vi "Load Commiunication Error.vi"(8 "error in (no error)":errorcluster, 11 "main ref":T1) -> (0 "error out":errorcluster)   [LabVIEW 2025]
uses:
  controls/LAB-IQ UI Data.ctl
  Traction Loop/Traction Receipe Enum.ctl
  <vilib>/Analysis/baseanly.llb/Mean (DBL).vi
  <vilib>/Analysis/NI_AALBase.lvlib
panel:
  out "Load Comflg":bool
  out "OLD VAL":dbl
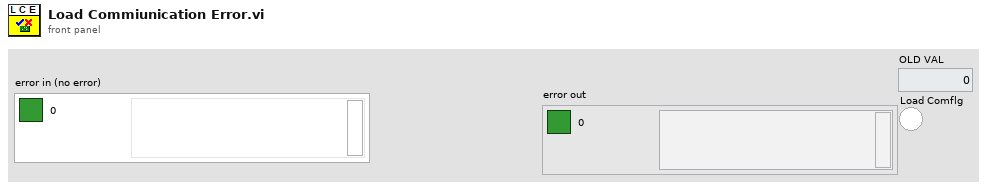
[diagram p1: front panel]
types:
  T1 = typedef "LAB-IQ UI Data.ctl" = cluster{"Main Home Screen":cluster{"GUI":refnum<vi>, "Platform Settings":refnum<vi>, "Configure":refnum<vi>, "Home":refnum<vi>, "EXIT":refnum<vi>, "service 2":refnum<vi>, "MainPage":refnum<vi>, "Analysis":refnum<vi>}, "Platform Settings":cluster{"mm/s  Surge":refnum<vi>, "Update Surge Speed":refnum<vi>, "Drive Error":refnum<vi>, "Disable Axis Jog Soft Limits":refnum<vi>, "mm/s  Sway":refnum<vi>, "Sway and Surge COM Status":refnum<vi>, "Heave COM Status":refnum<vi>, "Enable Platform":refnum<vi>, "Surge Forward Main":refnum<vi>, "Sway Right Main":refnum<vi>, "Sway Left Main":refnum<vi>, "Heave Down Main":refnum<vi>, "Heave Up main":refnum<vi>, "Update Sway Speed":refnum<vi>, "Update Heave Speed":refnum<vi>, "mm/s Heave":refnum<vi>, "mm/sec":refnum<vi>, "mm":refnum<vi>, "Surge Backward Main":refnum<vi>}, "Analysis Screen":cluster{"Analysis Home":refnum<vi>, "Surface Analysis":refnum<vi>, "Imaging":refnum<vi>, "Image Analysis":refnum<vi>, "Post Analysis":refnum<vi>}, "Config Screen":cluster{"Select Load Head":refnum<vi>, "Notes :":refnum<vi>, "FILE":refnum<vi>, "Sample ID :":refnum<vi>, "Operator ID :":refnum<vi>, "Operator Name :":refnum<vi>, "Auto":refnum<vi>}, "Motion Module":cluster{"zNL":refnum<vi>, "NL disp":refnum<vi>, "Rotary Tab":refnum<vi>, "Motion Direction:  3":refnum<vi>, "E.Velocity 2":refnum<vi>, "e.v/ssr 2":refnum<vi>, "Enter Fixed E.Velocity 2":refnum<vi>, "Enter Final SRR 2":refnum<vi>, "Enter initial SRR 2":refnum<vi>, "Enter Fixed SRR 2":refnum<vi>, "Enter the Final E.Velocity (m/s) 2":refnum<vi>, "Enter initial E.Velocity (m/s) 2":refnum<vi>, "Final Speed (RPM) 3":refnum<vi>, "Initial Speed (RPM) 2":refnum<vi>, "Enter the Final Velocity (m/s) 3":refnum<vi>, "Enter initial Velocity (m/s)  3":refnum<vi>, "Ramp Up 2":refnum<vi>, "TEST SELECTION":refnum<vi>, "SPEED SELECTION : ":refnum<vi>, "Angular Oscillation Set":refnum<vi>, "Traction":refnum<vi>, "Step Speed":refnum<vi>, "StepTable For Load-Speed":refnum<vi>, "StepTable For Speed":refnum<vi>, "Surge Forward MM":refnum<vi>, "Surge Backward MM":refnum<vi>, "M3 Image":refnum<vi>, "String 39":refnum<vi>, "Sway Left MM":refnum<vi>, "Sway Right MM":refnum<vi>, "Disable Axis Jog Soft Limits":refnum<vi>, "mm":refnum<vi>, "Heave Down MM":refnum<vi>, "Heave Up MM":refnum<vi>, "Wear Track Diameter (mm)":refnum<vi>, "Set WTD":refnum<vi>, "HomeScratch":refnum<vi>, "HomeRot":refnum<vi>, "PlaceModule":refnum<vi>, "Enter the Angle (Deg)":refnum<vi>, "Enter the Frequency (Hz)":refnum<vi>, "Motion Mode:":refnum<vi>, "LR Sway":refnum<vi>, "Rot Hor":refnum<vi>, "Scratch":refnum<vi>, "LR Cam":refnum<vi>, "MMBack":refnum<vi>, "MMNext":refnum<vi>, "Rot Ver":refnum<vi>, "Rotary Module Selection":refnum<vi>, "calculate rotary":refnum<vi>, "SPEED SELECTION : rotary":refnum<vi>, "Import 2":refnum<vi>, "Save 2":refnum<vi>, "File Path :  2":refnum<vi>, "String 45":refnum<vi>, "StepTable For Speed 3":refnum<vi>, "Enter the Speed(mm/sec)":refnum<vi>, "Enter the Speed(RPM)":refnum<vi>, "Enter Scratch Speed (mm/s):":refnum<vi>, "SwaySpeed Set":refnum<vi>, "Scartch Offset":refnum<vi>, "Motion type:":refnum<vi>, "HomeScratch 2":refnum<vi>, "Enter Scratch length (mm):":refnum<vi>, "Wear Track Diameter":refnum<vi>, "Rotary Speed Exced":refnum<vi>, "Scratch Mode":refnum<vi>, "No of Scratch":refnum<vi>}, "Environmental control":cluster{"Humidity  Status  3":refnum<vi>, "Low Temp  Status  2":refnum<vi>, "TK4 status 2":refnum<vi>, "Stage Temperature":refnum<vi>, "Sample Temperature":refnum<vi>, "Humidity (Amb)":refnum<vi>, "Clear List":refnum<vi>, "Add to list":refnum<vi>, "Wear":refnum<vi>, "Vibration":refnum<vi>, "Humidity (Chamber)":refnum<vi>, "Temperature (Chamber)":refnum<vi>, "ECR ":refnum<vi>, "Temperature (Amb)":refnum<vi>, "Microphone":refnum<vi>, "Acoustic Emission 3":refnum<vi>, "SNext":refnum<vi>, "APBack":refnum<vi>, "Enter the Temperature (°C):":refnum<vi>, "Enter the Stage \nTemperature (°C):":refnum<vi>, "Enter the Humidity (%Rh):":refnum<vi>, "Low Temp":refnum<vi>, "High Temp":refnum<vi>, "Humidity":refnum<vi>, "Sensors Picked":refnum<vi>}, "About Screen":cluster{"Password":refnum<vi>, "Home Service":refnum<vi>, "Advanced Setting":refnum<vi>, "About Tab":refnum<vi>, "ECR Port:":refnum<vi>, "Ramp Port:":refnum<vi>, "Installation/Replacement completed":refnum<vi>, "Loahead":refnum<vi>, "Heave and Surge COM Port:":refnum<vi>, "Sway COM Port:":refnum<vi>, "Temp Modbus:":refnum<vi>, "Humidity Port:":refnum<vi>, "Edit Gain Constants":refnum<vi>, "Save Gain Constants":refnum<vi>}, "Main Screen":cluster{"Main Screen Tab":refnum<vi>, "Angle and Frequency":refnum<vi>, "Stroke (mm)":refnum<vi>, "Angle (Deg)":refnum<vi>, "Main Speed Tab":refnum<vi>, "MTM MOTOR DISPLAY":refnum<vi>, "Disc Speed (m/sec)":refnum<vi>, "Ball Speed (m/sec)":refnum<vi>, "Disc Speed (RPM)":refnum<vi>, "Ball Speed (RPM)":refnum<vi>, "SPEED TAB":refnum<vi>, "Speed (m/sec)":refnum<vi>, "Set Speed (m/sec)":refnum<vi>, "Speed (RPM)":refnum<vi>, "Set Speed":refnum<vi>, "Time Tab":refnum<vi>, "Time ( HH:MM:SS ) 2":refnum<vi>, "Test Duration":refnum<vi>, "Test Duration 4":refnum<vi>, "TEST CYCLE":refnum<vi>, "TOTAL CYCLES":refnum<vi>, "Set Load (N)":refnum<vi>, "Temp Tabs":refnum<vi>, "Heater":refnum<vi>, "TK4 status":refnum<vi>, "ChamberTemp":refnum<vi>, "SetTmp":refnum<vi>, "Controller  Status":refnum<vi>, "ChamberTemp 2":refnum<vi>, "SetTmp 2":refnum<vi>, "Controller  Status 2":refnum<vi>, "ChamberTemp 3":refnum<vi>, "SetTmp 3":refnum<vi>, "Cooling":refnum<vi>, "Load Communication":refnum<vi>, "Ambient \nTemperature":refnum<vi>, "HumCOMStatus":refnum<vi>, "Ambient\n Humidity":refnum<vi>, "Freq (Hz)":refnum<vi>, "Load En":refnum<vi>, "NLt":refnum<vi>, "zNL 2":refnum<vi>, "Humidity On":refnum<vi>, "humidity disp":refnum<vi>, "Set Humidity":refnum<vi>, "NL disp 2":refnum<vi>, "Humidity On 2":refnum<vi>, "humidity disp 2":refnum<vi>, "Set Humidity 2":refnum<vi>, "NL disp 3":refnum<vi>, "AppLoadSeq scratch":refnum<vi>, "Stop Scratch":refnum<vi>, "ClrLog":refnum<vi>, "Trip Log":refnum<vi>, "STOP":refnum<vi>, "Start Test":refnum<vi>, "Test status":refnum<vi>, "AR Led":refnum<vi>, "Data":refnum<vi>, "Health":refnum<vi>, "Sway COM Status":refnum<vi>, "Heave COM Status":refnum<vi>, "Grp Tab":refnum<vi>, "Sub Graph":refnum<vi>, "SD (mm)":refnum<vi>, "Siliding distance Reset Graph":refnum<vi>, "SDGp":refnum<vi>, "Humidity Reset Graph":refnum<vi>, "HumrGp":refnum<vi>, "Acoustic Emission (mV)":refnum<vi>, "Aqucostic Reset Graph":refnum<vi>, "gACQUOS":refnum<vi>, "ECR RESET":refnum<vi>, "ECR":refnum<vi>, "Temperature Reset":refnum<vi>, "Acoustic Emission (mV) 2":refnum<vi>, "Aqucostic Reset Graph 2":refnum<vi>, "gACQUOS 2":refnum<vi>, "ECR RESET 2":refnum<vi>, "ECR 2":refnum<vi>, "Temperature Reset 2":refnum<vi>, "Temperature (deg c)":refnum<vi>, "Speed Reset Graph":refnum<vi>, "Speed Tab":refnum<vi>, "MTM DISC  SPEED":refnum<vi>, "MTM BALL SPEED":refnum<vi>, "speed mm/sec":refnum<vi>, "Hymidity":refnum<vi>, "Humidity Disable trip":refnum<vi>, "CoF Trip  2":refnum<vi>, "Depth Trip":refnum<vi>, "Weart Deapth":refnum<vi>, "Depth Reset Graph":refnum<vi>, "Weart":refnum<vi>, "Depthz":refnum<vi>, "Depth (µm)":refnum<vi>, "WearGp":refnum<vi>, "NL Trip 2":refnum<vi>, "Load pid":refnum<vi>, "Load Disable Trip":refnum<vi>, "Load Reset Graph":refnum<vi>, "NL Display 4":refnum<vi>, "Main Chart 3":refnum<vi>, "BACK":refnum<vi>, "Depth Trip 2":refnum<vi>, "COF TRIP ":refnum<vi>, "Friction Force (N)":refnum<vi>, "FF Reset Graph":refnum<vi>, "FF Disable Trip":refnum<vi>, "FF TRIP":refnum<vi>, "COF Disable Trip":refnum<vi>, "COF Reset Graph":refnum<vi>, "Start Test Temp":refnum<vi>, "zFF":refnum<vi>, "Friction Force (N) Graph":refnum<vi>, "Coefficient of Friction":refnum<vi>, "Scratch Start Test":refnum<vi>, "FF Tab":refnum<vi>, "Cyclic Friction Force (N)":refnum<vi>, "CZ FF":refnum<vi>, "Cyclic Friction Force (N) Graph":refnum<vi>, "Cyclic Coefficient of Friction":refnum<vi>, "Cyclic FF TRIP":refnum<vi>, "Cyclic FF Disable Trip":refnum<vi>, "cyclic COF Disable Trip":refnum<vi>, "cyclic COF TRIP":refnum<vi>, "cyclic COF Reset Graph":refnum<vi>, "Cyclic FF Reset Graph":refnum<vi>, "Test Trip":refnum<vi>, "Multi Scratch Pass":refnum<vi>, "Scratch Start Recording":refnum<vi>}, "Loading":cluster{"Indentation":refnum<vi>, "Reference Sample":refnum<vi>, "Load Cell Communication Slide":refnum<vi>, "com 3":refnum<vi>, "com":refnum<vi>, "DecaForce COM Status":refnum<vi>, "Update":refnum<vi>, "Clear 3":refnum<vi>, "seq":refnum<vi>, "Stribeck table":refnum<vi>, "Stribeck Table  For loading":refnum<vi>, "Loading Mode":refnum<vi>, "Enter the Final Load (N)":refnum<vi>, "Enter the CoF Trip":refnum<vi>, "Enter the Friction Force Trip":refnum<vi>, "Enter the Normal load Trip":refnum<vi>, "Enter the Load  (N)":refnum<vi>, "KiloForce":refnum<vi>, "DecaForce ":refnum<vi>, "MicroForce":refnum<vi>, "LHBack":refnum<vi>, "LHNext":refnum<vi>, "Enter the Loading Rate (N/min)":refnum<vi>, "Message":refnum<vi>, "Warning 2":refnum<vi>, "SSP 0.75":refnum<vi>, "SSP 0.5":refnum<vi>, "SSP 0.3":refnum<vi>, "Warning":refnum<vi>, "gui GIF":refnum<vi>, "Communication is established":refnum<vi>, "AppLoad 4":refnum<vi>, "Multipoint":refnum<vi>, "Load Selection":refnum<vi>}, "PID":cluster{"Ramp MulFac":refnum<vi>, "pulses LoadDiffRamp(2..10)":refnum<vi>, "PulseControlRamp(diff<=3N)":refnum<vi>, "SetLoadDeadband(%) Load(0-10N)":refnum<vi>, "PID gains out delay (microForce)":refnum<vi>, "Ramp":refnum<vi>, "Gain 2":refnum<vi>, "pulses LoadDiff(2..10)":refnum<vi>, "pulses LoadDiff(11..50)":refnum<vi>, "PulseControl(diff<=3N)":refnum<vi>, "SetLoadDeadband(%)  2":refnum<vi>, "Dummy Run":refnum<vi>, "Vertical load (N)":refnum<vi>, "AutoTune":refnum<vi>, "Offset 3 ":refnum<vi>, "apply load":refnum<vi>, "Offset  3":refnum<vi>, "apply load 2":refnum<vi>, "Enter ByPass Load":refnum<vi>, "reinit 3":refnum<vi>, "output range delay":refnum<vi>, "PID gains out delay":refnum<vi>, "Bypass Load":refnum<vi>, "pulsesSent":refnum<vi>, "pulses ":refnum<vi>, "actpid":refnum<vi>, "gFF Rot":refnum<vi>, "pulses LoadDiff(21..1000)":refnum<vi>, "Delay":refnum<vi>, "deadband":refnum<vi>}, "Config Parameters":cluster{"Tab Control 3":refnum<vi>, "Tab Control 19":refnum<vi>, "SAMPLES":refnum<vi>, "Re-initilaize":refnum<vi>, "Filter ON/OFF":refnum<vi>, "TracHomeSurgeOffsetCounts 10MM":refnum<vi>, "TracHomeSwayOffsetCounts 10MM":refnum<vi>, "Acoustic Emission:":refnum<vi>, "Apply Filter (FF)":refnum<vi>, "Filter% 2":refnum<vi>, "Apply Filter (Load)":refnum<vi>, "Filter% ":refnum<vi>, "Sway distance (mm)":refnum<vi>, "Surge distance (mm)":refnum<vi>, "DataSavingLoopDelay(ms)":refnum<vi>, "SAVE 2":refnum<vi>, "Enter Distance":refnum<vi>, "Sway Counts:":refnum<vi>, "Distance (mm): 3":refnum<vi>, "Surge Counts:":refnum<vi>, "Distance (mm): 2":refnum<vi>, "Distance (mm):":refnum<vi>, "Heave Counts:":refnum<vi>, "LRMHomeSurgeOffsetCounts":refnum<vi>, "LRMHomeSwayOffsetCounts":refnum<vi>, "TracHomeSurgeOffsetCounts 20MM":refnum<vi>, "TracHomeSwayOffsetCounts 20MM":refnum<vi>, "RotHomeSwayOffsetCounts":refnum<vi>, "RotHomeSurgeOffsetCounts":refnum<vi>, "Heave distance":refnum<vi>, "Zmm":refnum<vi>, "Heave Pulses/mm":refnum<vi>, "Surge Pulses/mm":refnum<vi>, "Sway Pulses/mm":refnum<vi>, "Heave Pitch":refnum<vi>, "Surge Pitch":refnum<vi>, "Sway Pitch":refnum<vi>, "Heave PPR":refnum<vi>, "Surge PPR":refnum<vi>, "Sway PPR":refnum<vi>, "Tab Control 5":refnum<vi>, "Tab Control 14":refnum<vi>, "Tab Control 26":refnum<vi>, "AE":refnum<vi>, "Heave Loop Delay":refnum<vi>, "Heave PID Speed":refnum<vi>, "Surge Jog Speed":refnum<vi>, "Heave Jog Speed":refnum<vi>, "Sway Loop Delay":refnum<vi>, "Sway PID Speed":refnum<vi>, "Sway Jog Speed":refnum<vi>, "DEPTH TRIP VALUE":refnum<vi>, "LOAD TRIP VALUE":refnum<vi>, "DEPTH TRIP   ENABLE":refnum<vi>, "LOAD TRIP  ENABLE":refnum<vi>, "CYCLIC FF TRIP VALUE":refnum<vi>, "FF TRIP VALUE":refnum<vi>, "CYCLIC CoF TRIP VALUE":refnum<vi>, "COF TRIP VALUE":refnum<vi>, "CYCLIC COF TRIP  ENABLE":refnum<vi>, "CYCLIC FF TRIP  ENABLE":refnum<vi>, "FF TRIP  ENABLE":refnum<vi>, "COF TRIP  ENABLE":refnum<vi>, "JOG TRIP LOAD VALUE (N)":refnum<vi>}, "Loading Com Port":cluster{"ClearAll":refnum<vi>, "Mz(Nm)":refnum<vi>, "My(Nm)":refnum<vi>, "Mx(Nm)":refnum<vi>, "Save Dwell":refnum<vi>, "Mx ":refnum<vi>, "My ":refnum<vi>, "Mz":refnum<vi>, "Fx(N)":refnum<vi>, "Fy(N)":refnum<vi>, "Fz(N)":refnum<vi>, "ZeroAll":refnum<vi>, "Acq Delay (ms)":refnum<vi>, "Burst Delay (ms)":refnum<vi>, "model":refnum<vi>, "SN":refnum<vi>, "FFx(N)":refnum<vi>, "Sensor IP":refnum<vi>, "Port":refnum<vi>, "FFy(N)":refnum<vi>, "Load(N)":refnum<vi>, "delete Handle":refnum<vi>, "Create Handle":refnum<vi>, "ft_data":refnum<vi>, "ft_range":refnum<vi>, "ft_data 2":refnum<vi>, "stop 6":refnum<vi>, "running_flag":refnum<vi>, "ft_udp_handle":refnum<vi>, "get-data-return":refnum<vi>, "get-range-return":refnum<vi>, "zero-return":refnum<vi>, "filter-return":refnum<vi>, "initial-return":refnum<vi>, "deleteHandle-result":refnum<vi>, "Load Cell Temp":refnum<vi>, "Load Cell":refnum<vi>}, "Heave AND Surge":cluster{"SURGE POSE":refnum<vi>, "error out Read":refnum<vi>, "HEAVE POSE":refnum<vi>, "State":refnum<vi>, "Homed":refnum<vi>, "Sequence ID":refnum<vi>, "error out Write":refnum<vi>, "faultCode":refnum<vi>, "Ack ID":refnum<vi>, "SPEED":refnum<vi>, "Distance":refnum<vi>, "Mode Command":refnum<vi>, "Heave and Surge Read":refnum<vi>, "Read Heave Temp":refnum<vi>, "Spare 15":refnum<vi>, "Spare 14":refnum<vi>, "Spare 13":refnum<vi>, "Spare 12":refnum<vi>, "Spare 11":refnum<vi>, "Spare 10":refnum<vi>, "Spare 9":refnum<vi>, "Spare 8":refnum<vi>, "Spare 7":refnum<vi>, "Spare 6":refnum<vi>, "Spare 5":refnum<vi>, "Spare 4":refnum<vi>, "Spare 2":refnum<vi>, "Spare 1":refnum<vi>, "Node Id":refnum<vi>, "Spare 3":refnum<vi>, "SPARE 4":refnum<vi>, "SPARE 3":refnum<vi>, "SPARE 2":refnum<vi>, "SPARE 1":refnum<vi>, "fwMajor":refnum<vi>, "fwMinor":refnum<vi>, "Manual Write":refnum<vi>, "Heave and Surge Write":refnum<vi>, "SPARE 5":refnum<vi>, "Reserved ":refnum<vi>, "SPARE 8":refnum<vi>, "SPARE 6":refnum<vi>, "SPARE 7":refnum<vi>, "SPARE 17":refnum<vi>, "SPARE 16":refnum<vi>, "SPARE 15":refnum<vi>, "SPARE 14":refnum<vi>, "SPARE 13":refnum<vi>, "SPARE 12":refnum<vi>, "SPARE 11":refnum<vi>, "SPARE 10":refnum<vi>, "SPARE 9":refnum<vi>, "System UPTIME":refnum<vi>, "Missed Packets":refnum<vi>, "faultCode Surge Right":refnum<vi>, "faultCode Surge Left":refnum<vi>, "faultCode Heave":refnum<vi>, "UPLINK HEAVE":refnum<vi>, "DOWNLINK HEAVE":refnum<vi>}, "New PID LOGIC":cluster{"Fine Tune Zone":refnum<vi>, "PID SDelay":refnum<vi>, "Max_pos_limit":refnum<vi>, "Min_pos_limit":refnum<vi>, "i_limit":refnum<vi>, "pct_scale":refnum<vi>, "Deadband":refnum<vi>, "Kd":refnum<vi>, "Ki":refnum<vi>, "Kp":refnum<vi>, "Current Position":refnum<vi>, "Set Load":refnum<vi>, "Current Load":refnum<vi>, "Pulse delta":refnum<vi>, "Init Step":refnum<vi>, "Max Step Linit":refnum<vi>, "min_deadband_floor":refnum<vi>, "dynamic_spindle_noise_scalar":refnum<vi>, "min_finetune_floor":refnum<vi>, "filter_alpha":refnum<vi>, "PID":refnum<vi>}, "SWAY ":cluster{"fwMajor":refnum<vi>, "Homed":refnum<vi>, "Rotary POSE":refnum<vi>, "State":refnum<vi>, "SWAY POSE":refnum<vi>, "Ack ID":refnum<vi>, "faultCode":refnum<vi>, "Node Id":refnum<vi>, "fwMinor":refnum<vi>, "Spare 6":refnum<vi>, "Spare 5":refnum<vi>, "Spare 4":refnum<vi>, "Spare 3":refnum<vi>, "Spare 2":refnum<vi>, "Spare 1":refnum<vi>, "Spare 7":refnum<vi>, "SPARE  5":refnum<vi>, "error out Write  SWAY ":refnum<vi>, "error out Read SWAY ":refnum<vi>, "Manual Write SWAY ":refnum<vi>, "SWAY WRITE":refnum<vi>, "SPARE  4":refnum<vi>, "SPARE  3":refnum<vi>, "SPARE 2":refnum<vi>, "SPARE 1":refnum<vi>, "Spare 15":refnum<vi>, "Spare 14":refnum<vi>, "Spare 13":refnum<vi>, "Spare 12":refnum<vi>, "Spare 11":refnum<vi>, "Spare 9":refnum<vi>, "Spare 8":refnum<vi>, "SPEED":refnum<vi>, "Distance":refnum<vi>, "Mode Command":refnum<vi>, "Sequence ID":refnum<vi>, "SWAY READ":refnum<vi>, "Spare 10":refnum<vi>, "Read SWAY Temp":refnum<vi>, "faultCode Sway ":refnum<vi>, "Missed Packets":refnum<vi>, "System UPTIME sway":refnum<vi>, "SPARE 6":refnum<vi>, "SPARE 7":refnum<vi>, "SPARE 9":refnum<vi>, "SPARE 11":refnum<vi>, "SPARE 10":refnum<vi>, "SPARE 8":refnum<vi>, "SPARE 13":refnum<vi>, "SPARE 12":refnum<vi>, "SPARE 17":refnum<vi>, "SPARE 16":refnum<vi>, "SPARE 15":refnum<vi>, "SPARE 14":refnum<vi>, "Reserved":refnum<vi>, "faultCode Rotary":refnum<vi>, "UPLINK SWAY":refnum<vi>, "DOWNLINK SWAY":refnum<vi>}, "Analysis Screen":cluster{"Analysis Home":refnum<vi>, "Refresh 2":refnum<vi>, "MEAN 4":refnum<vi>, "SD 4":refnum<vi>, "VARIANCE 4":refnum<vi>, "MEAN  3":refnum<vi>, "SD  3":refnum<vi>, "VARIANCE  3":refnum<vi>, "MEAN 2":refnum<vi>, "SD  2":refnum<vi>, "VARIANCE 2":refnum<vi>, "MEAN":refnum<vi>, "SD":refnum<vi>, "VARIANCE":refnum<vi>, "File 4 Discription":refnum<vi>, "OPEN 4":refnum<vi>, "File Name 4":refnum<vi>, "OPEN 3":refnum<vi>, "File 3 Discription":refnum<vi>, "File Name 3":refnum<vi>, "Y-AXIS":refnum<vi>, "X-AXIS":refnum<vi>, "XY Graph":refnum<vi>, "File Name 2":refnum<vi>, "File Name 1":refnum<vi>, "OPEN 2":refnum<vi>, "OPEN 1":refnum<vi>, "File 1 Discription ":refnum<vi>, "File 2 Discription":refnum<vi>, "Export":refnum<vi>, "File Format":refnum<vi>}, "Traction":cluster{"faultCode Traction 2":refnum<vi>, "faultCode Traction 1":refnum<vi>, "Missed Packets":refnum<vi>, "System UPTIME Traction":refnum<vi>, "SPARE 17":refnum<vi>, "SPARE 16":refnum<vi>, "SPARE 15":refnum<vi>, "SPARE 14":refnum<vi>, "SPARE 13":refnum<vi>, "SPARE 12":refnum<vi>, "SPARE 11":refnum<vi>, "SPARE 10":refnum<vi>, "SPARE 9":refnum<vi>, "SPARE 8":refnum<vi>, "SPARE 7":refnum<vi>, "SPARE 6":refnum<vi>, "Reserved":refnum<vi>, "SPARE  5":refnum<vi>, "Manual Write TRACTION":refnum<vi>, "TRACTION WRITE":refnum<vi>, "SPARE  4":refnum<vi>, "SPARE  3":refnum<vi>, "SPARE 2":refnum<vi>, "SPARE 1":refnum<vi>, "Spare 7":refnum<vi>, "Spare 6":refnum<vi>, "Spare 5":refnum<vi>, "Spare 4":refnum<vi>, "Spare 2":refnum<vi>, "Spare 1":refnum<vi>, "Node Id":refnum<vi>, "Read TRACTION Temp":refnum<vi>, "fwMinor":refnum<vi>, "fwMajor":refnum<vi>, "faultCode":refnum<vi>, "TRACTION POSE":refnum<vi>, "TRACTION POSE 2":refnum<vi>, "Homed":refnum<vi>, "State":refnum<vi>, "Ack ID":refnum<vi>, "SPEED":refnum<vi>, "Distance":refnum<vi>, "Mode Command":refnum<vi>, "Sequence ID":refnum<vi>, "error out Read TRACTION":refnum<vi>, "error out Write  TRACTION":refnum<vi>, "TRACTION READ":refnum<vi>, "Spare 3":refnum<vi>, "Downlink traction":refnum<vi>, "Uplink Traction":refnum<vi>}, "Traction reciepe":cluster{"SRR Sweep Range (%) Stribeck":refnum<vi>, "Traction Receipe":refnum<vi>, "Total Execution Time":refnum<vi>, "Total Steps":refnum<vi>, "Duration / Step (s)  Stribeck":refnum<vi>, "STRIBECK Fixed SRR List (%)":refnum<vi>, "Duration / Step (s) Traction":refnum<vi>, "SRR Sweep Range (%) traction":refnum<vi>, "Rolling Speed (mm/s)":refnum<vi>, "Temperature Stages (°C)":refnum<vi>, "Ball Load (N)":refnum<vi>, "Lubricant Name":refnum<vi>, "Profile File Name":refnum<vi>, "SET entrainment Velocity":refnum<vi>, "Test Array Size":refnum<vi>, "SRR INDEX [ STRIBECK]":refnum<vi>, "Stribeck Size":refnum<vi>, "SET SRR":refnum<vi>, "ELAPSED TIMER ":refnum<vi>, "BALL SET RPM":refnum<vi>, "DISC SET RPM":refnum<vi>, "SET LOAD":refnum<vi>, "TEMPERATURE READ":refnum<vi>, "SET TEMPERATURE":refnum<vi>, "Traction Size":refnum<vi>, "DISC SPEED (rpm)":refnum<vi>, "BALL SPEED (rpm)":refnum<vi>, "BALL WEAR TRACK":refnum<vi>, "DISC WEARTRACK":refnum<vi>, "SRR INDEX [ TRACTION]":refnum<vi>, "Start Index Type":refnum<vi>, "Enum - Menu":refnum<vi>, "Ball (mm/sec)":refnum<vi>, "Disc (mm/sec)":refnum<vi>}, "Traction Control":cluster{"HomeTraction":refnum<vi>, "Demo Mode Display":refnum<vi>, "Traction Message":refnum<vi>, "Traction Step Update Details":refnum<vi>, "Main Tab sequence for selection":refnum<vi>, "Ramp Tab":refnum<vi>, "e.v/ssr":refnum<vi>, "Enter Fixed E.Velocity":refnum<vi>, "Enter Final SRR":refnum<vi>, "Enter initial SRR":refnum<vi>, "Enter Fixed SRR":refnum<vi>, "Enter the Final E.Velocity (m/s)":refnum<vi>, "Enter initial E.Velocity (m/s)":refnum<vi>, "Ball WTD":refnum<vi>, "E.Velocity":refnum<vi>, "Enter the Final Velocity (m/s)":refnum<vi>, "Enter initial Velocity (m/s)":refnum<vi>, "Ramp Up   Disc":refnum<vi>, "Initial DiscSpeed (RPM)":refnum<vi>, "Final Speed (RPM) Ball":refnum<vi>, "Final Speed (RPM)":refnum<vi>, "Initial Speed (RPM) Ball":refnum<vi>, "Enter the Final Velocity (m/s) Ball":refnum<vi>, "Enter initial Velocity (m/s) Ball":refnum<vi>, "Ramp Up":refnum<vi>, "ExceedBallSpeed step":refnum<vi>, "ExceedDiscSpeed":refnum<vi>, "BallSpeed Exceed Indication":refnum<vi>, "Apply":refnum<vi>, "SPEED SELECTION : MTM":refnum<vi>, "SPEED SELECTION : MTM 2":refnum<vi>, "TEST SELECTION (MTM)":refnum<vi>, "MTM Test Selection":refnum<vi>, "File Path Tab":refnum<vi>, "File Path String":refnum<vi>, "Save":refnum<vi>, "Save  2":refnum<vi>, "Import ":refnum<vi>, "File Path :":refnum<vi>, "Step Sequence Indication Tab":refnum<vi>, "Step Sequence Indication":refnum<vi>, "Calculate Step":refnum<vi>, "StepTable":refnum<vi>, "ExceedDiscSpeed  Cinstant Speed":refnum<vi>, "ExceedBallSpeed Constant":refnum<vi>, "TEST SELECTION (MTM) 2":refnum<vi>, "SPEED SELECTION : MTM 3":refnum<vi>, "MTM Test Selection 2":refnum<vi>, "Enter the Speed (m/sec): ":refnum<vi>, "Enter the Speed (m/sec):  2":refnum<vi>, "Enter the Speed (RPM):":refnum<vi>, "Lower Spped ":refnum<vi>, "Upper":refnum<vi>, "Enter the Speed (RPM):Ball":refnum<vi>, "Disc Motion Direction: ":refnum<vi>, "Ball Motion Direction :":refnum<vi>, "Motion Mode: ":refnum<vi>, "Wear Track Diameter (mm) ":refnum<vi>, "Disc Speed Indicator":refnum<vi>, "ExceedBallSpeed":refnum<vi>}, "Acquostic":cluster{"Last Config Rejected ":refnum<vi>, "rx command count":refnum<vi>, "Current Filter Id":refnum<vi>, "Isolated Gain":refnum<vi>, "DAQ Status":refnum<vi>, "error out":refnum<vi>, "error in (no error)":refnum<vi>, "Uplink Packet":refnum<vi>, "data out":refnum<vi>, "Downlink Packet":refnum<vi>, "Signal Energy":refnum<vi>, "Amplitude db_AE":refnum<vi>, "Peak Amplitude":refnum<vi>, "AE Ring-Down Counts":refnum<vi>, "Gains":refnum<vi>, "Manual Write Acquostic":refnum<vi>}}
  T2 = enum8{"Enabled", "Disabled", "Disabled and Grayed Out"}
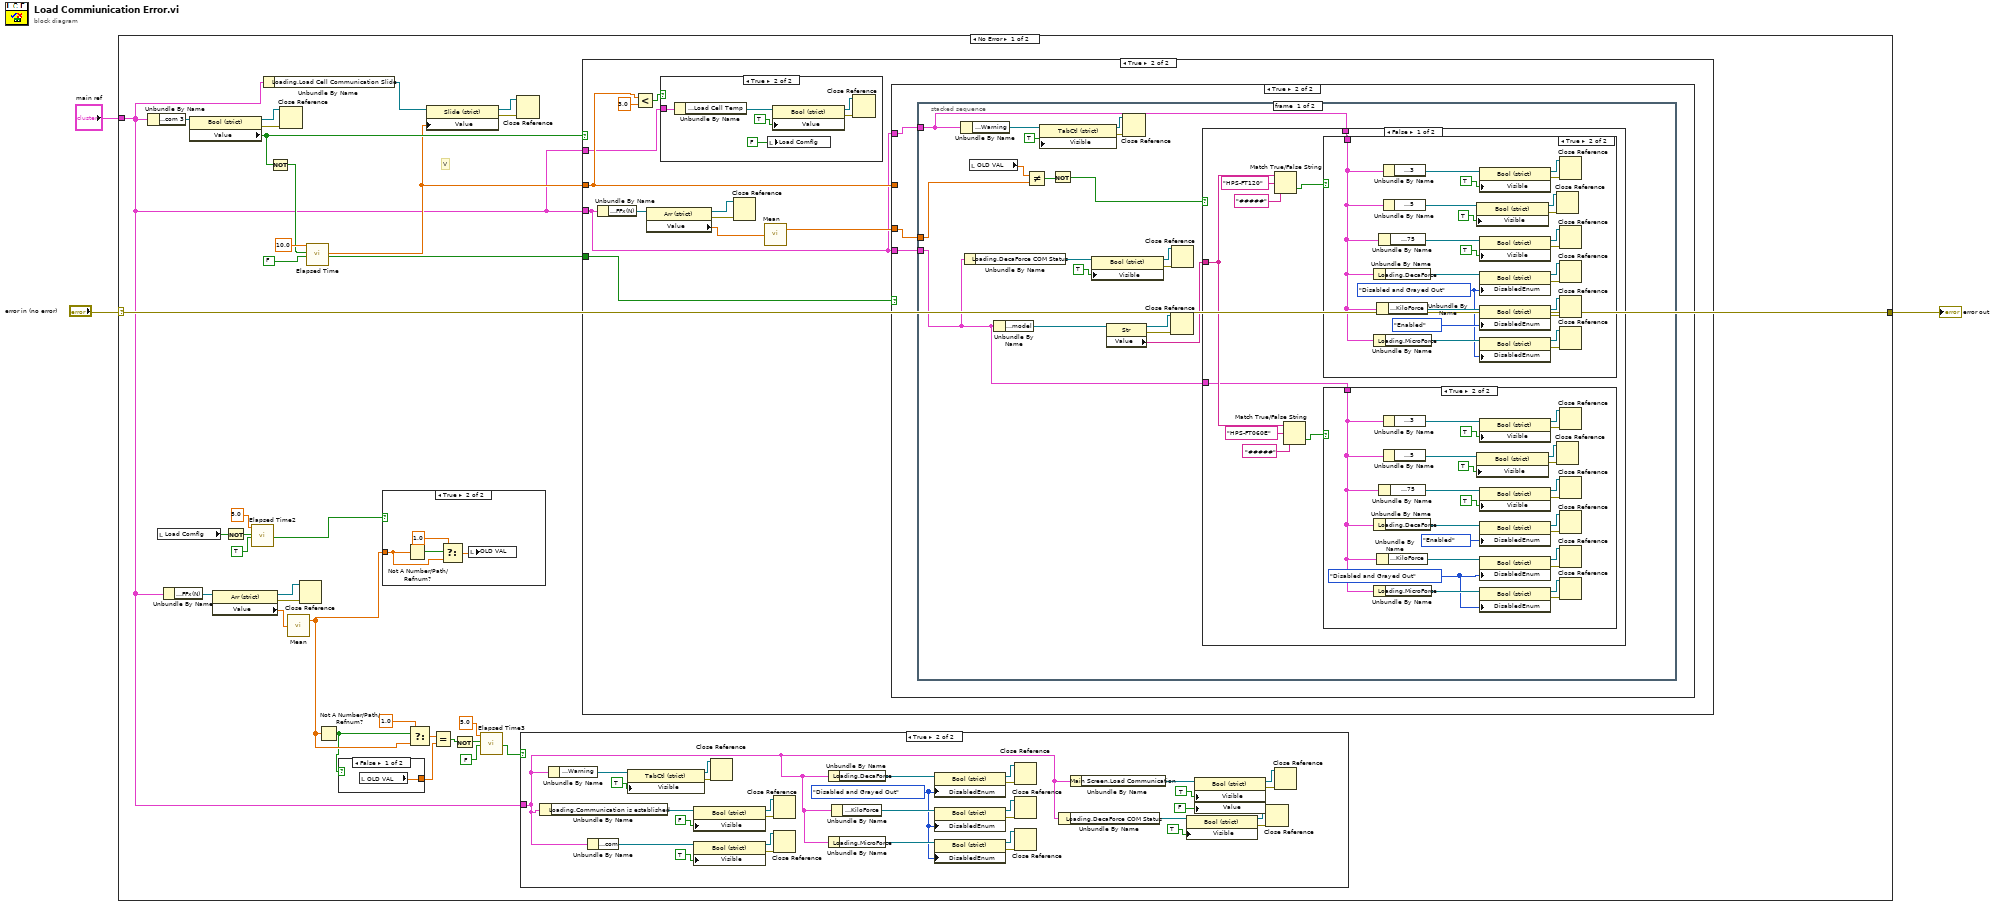
[diagram p0: block diagram]
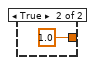
[diagram p2: hidden frame]
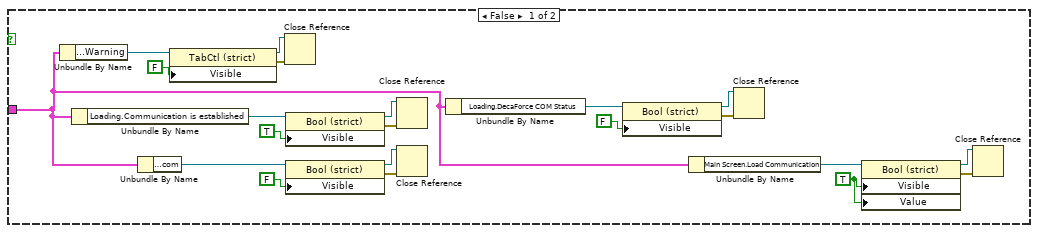
[diagram p3: hidden frame]
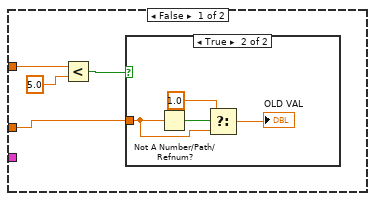
[diagram p7: hidden frame]
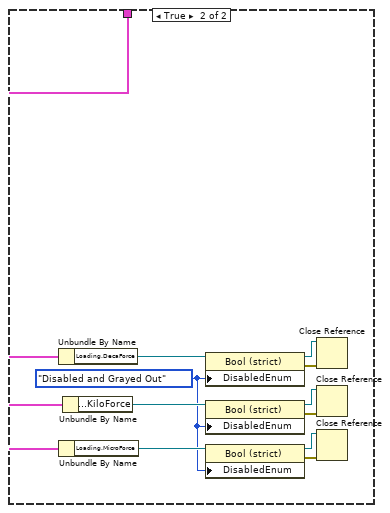
[diagram p11: hidden frame]
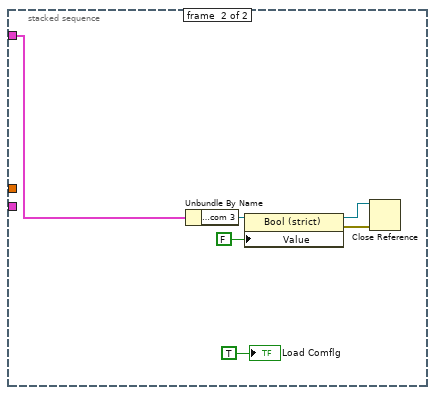
[diagram p12: hidden frame]
diagram:
  n1 = case shown="No Error" "error in (no error)" {
    selector: "error in (no error)" -> [w35 _]
    tunnel: "main ref" -> [w5 _]
    tunnel: [w35 _] -> w1
    frame No Error {
      # "V"
      n2 = Unbundle By Name(w5) -> ("Loading.com 3"=w36:refnum<vi>)
      n3 = local read "Load Comflg"() -> (w23:bool)
      n4 = Unbundle By Name(w5) -> ("Loading Com Port.FFx(N)"=w16:refnum<vi>)
      n5 = property class="Bool (strict)"(reference=w36) -> (reference out=w33:refnum<vi>, error out=w34:errorcluster, "Value"=w31:bool)  [unwired: 1 in]
      n6 = property class="Arr (strict)"(reference=w16) -> (reference out=w18:refnum<vi>, error out=w17:errorcluster, "Value"=w19:dbl[])  [unwired: 1 in]
      n7 = Not(x=w23) -> (.not. x?=w22:bool)
      n8 = call "Elapsed Time2"("Time Target (s)"=5.0, "Reset"=w22, "Auto Reset"=TRUE) -> ("Time has Elapsed"=w15:bool)  [unwired: 9 in, 7 out]
      n9 = Unbundle By Name(w5) -> ("Loading.Load Cell Communication Slide"=w28:refnum<vi>)
      n10 = Not(x=w31) -> (.not. x?=w30:bool)
      n11 = Close Reference(reference=w33, error in (no error)=w34) -> ()  [unwired: 1 out]
      n12 = call-poly <vilib>:"Mean.vi"("X"=w19) -> ("mean"=w13:dbl)  [unwired: 1 out]
      n13 = Close Reference(reference=w18, error in (no error)=w17) -> ()  [unwired: 1 out]
      n14 = call "Elapsed Time"("Time Target (s)"=10.0, "Reset"=w30, "Auto Reset"=FALSE) -> ("Elapsed Time (s)"=w24:dbl, "Time has Elapsed"=w25:bool)  [unwired: 9 in, 6 out]
      n15 = Not A Number/Path/Refnum?(number/path/refnum=w13) -> (NaN/Path/Refnum?=w4:bool)
      n16 = case shown="False" w4 {
        tunnel: [w37 1.0 ("OLD VAL")] -> w11
        frame False {
          n17 = local read "OLD VAL"() -> (w37:dbl)
        }
        frame True {
        }
      }
      n18 = case shown="True" w15 {
        tunnel: w13 -> [_ w93]
        frame False {
        }
        frame True {
          n19 = Not A Number/Path/Refnum?(number/path/refnum=w93) -> (NaN/Path/Refnum?=w95:bool)
          n20 = Select(t=1.0, s=w95, f=w93) -> (s? t:f=w92:dbl)
          n21 = local write "OLD VAL"(w92) -> ()
        }
      }
      n22 = Select(t=1.0, s=w4, f=w13) -> (s? t:f=w12:dbl)
      n23 = property class="Slide (strict)"(reference=w28, "Value"=w24) -> (reference out=w26:refnum<vi>, error out=w27:errorcluster)  [unwired: 1 in]
      n24 = Equal?(x=w12, y=w11) -> (x = y?=w7:bool)
      n25 = Not(x=w7) -> (.not. x?=w8:bool)
      n26 = call "Elapsed Time3"("Time Target (s)"=5.0, "Reset"=w8, "Auto Reset"=FALSE) -> ("Time has Elapsed"=w6:bool)  [unwired: 9 in, 7 out]
      n27 = Close Reference(reference=w26, error in (no error)=w27) -> ()  [unwired: 1 out]
      n28 = case shown="True" w6 {
        tunnel: w5 -> [w40 w61]
        frame False {
          w39 = TRUE ("Visible")
          n29 = Unbundle By Name(w40) -> ("Loading.Warning"=w59:refnum<vi>)
          n30 = Unbundle By Name(w40) -> ("Loading.Communication is established"=w53:refnum<vi>)
          n31 = Unbundle By Name(w40) -> ("Loading.com"=w52:refnum<vi>)
          n32 = property class="TabCtl (strict)"(reference=w59, "Visible"=FALSE) -> (reference out=w57:refnum<vi>, error out=w58:errorcluster)  [unwired: 1 in]
          n33 = Close Reference(reference=w57, error in (no error)=w58) -> ()  [unwired: 1 out]
          n34 = property class="Bool (strict)"(reference=w53, "Visible"=TRUE) -> (reference out=w48:refnum<vi>, error out=w54:errorcluster)  [unwired: 1 in]
          n35 = property class="Bool (strict)"(reference=w52, "Visible"=FALSE) -> (reference out=w49:refnum<vi>, error out=w51:errorcluster)  [unwired: 1 in]
          n36 = Close Reference(reference=w48, error in (no error)=w54) -> ()  [unwired: 1 out]
          n37 = Close Reference(reference=w49, error in (no error)=w51) -> ()  [unwired: 1 out]
          n38 = Unbundle By Name(w40) -> ("Loading.DecaForce COM Status"=w47:refnum<vi>)
          n39 = property class="Bool (strict)"(reference=w47, "Visible"=FALSE) -> (reference out=w45:refnum<vi>, error out=w46:errorcluster)  [unwired: 1 in]
          n40 = Unbundle By Name(w40) -> ("Main Screen.Load Communication"=w41:refnum<vi>)
          n41 = Close Reference(reference=w45, error in (no error)=w46) -> ()  [unwired: 1 out]
          n42 = property class="Bool (strict)"(reference=w41, "Visible"=w39, "Value"=w39) -> (reference out=w43:refnum<vi>, error out=w42:errorcluster)  [unwired: 1 in]
          n43 = Close Reference(reference=w43, error in (no error)=w42) -> ()  [unwired: 1 out]
        }
        frame True {
          w71 = T2."Disabled and Grayed Out" ("Disabled")
          n44 = Unbundle By Name(w61) -> ("Loading.Communication is established"=w84:refnum<vi>)
          n45 = Unbundle By Name(w61) -> ("Loading.Warning"=w91:refnum<vi>)
          n46 = Unbundle By Name(w61) -> ("Loading.com"=w83:refnum<vi>)
          n47 = property class="TabCtl (strict)"(reference=w91, "Visible"=TRUE) -> (reference out=w89:refnum<vi>, error out=w90:errorcluster)  [unwired: 1 in]
          n48 = property class="Bool (strict)"(reference=w84, "Visible"=FALSE) -> (reference out=w86:refnum<vi>, error out=w85:errorcluster)  [unwired: 1 in]
          n49 = property class="Bool (strict)"(reference=w83, "Visible"=TRUE) -> (reference out=w70:refnum<vi>, error out=w82:errorcluster)  [unwired: 1 in]
          n50 = Close Reference(reference=w89, error in (no error)=w90) -> ()  [unwired: 1 out]
          n51 = Close Reference(reference=w86, error in (no error)=w85) -> ()  [unwired: 1 out]
          n52 = Close Reference(reference=w70, error in (no error)=w82) -> ()  [unwired: 1 out]
          n53 = Unbundle By Name(w61) -> ("Loading.DecaForce"=w80:refnum<vi>)
          n54 = Unbundle By Name(w61) -> ("Loading.MicroForce"=w75:refnum<vi>)
          n55 = Unbundle By Name(w61) -> ("Loading.KiloForce"=w77:refnum<vi>)
          n56 = property class="Bool (strict)"(reference=w80, "DisabledEnum"=w71) -> (reference out=w72:refnum<vi>, error out=w79:errorcluster)  [unwired: 1 in]
          n57 = property class="Bool (strict)"(reference=w77, "DisabledEnum"=w71) -> (reference out=w76:refnum<vi>, error out=w78:errorcluster)  [unwired: 1 in]
          n58 = property class="Bool (strict)"(reference=w75, "DisabledEnum"=w71) -> (reference out=w73:refnum<vi>, error out=w74:errorcluster)  [unwired: 1 in]
          n59 = Close Reference(reference=w72, error in (no error)=w79) -> ()  [unwired: 1 out]
          n60 = Close Reference(reference=w76, error in (no error)=w78) -> ()  [unwired: 1 out]
          n61 = Close Reference(reference=w73, error in (no error)=w74) -> ()  [unwired: 1 out]
          n62 = Unbundle By Name(w61) -> ("Loading.DecaForce COM Status"=w69:refnum<vi>)
          n63 = Unbundle By Name(w61) -> ("Main Screen.Load Communication"=w63:refnum<vi>)
          n64 = property class="Bool (strict)"(reference=w69, "Visible"=TRUE) -> (reference out=w67:refnum<vi>, error out=w68:errorcluster)  [unwired: 1 in]
          n65 = property class="Bool (strict)"(reference=w63, "Visible"=TRUE, "Value"=FALSE) -> (reference out=w65:refnum<vi>, error out=w64:errorcluster)  [unwired: 1 in]
          n66 = Close Reference(reference=w67, error in (no error)=w68) -> ()  [unwired: 1 out]
          n67 = Close Reference(reference=w65, error in (no error)=w64) -> ()  [unwired: 1 out]
        }
      }
      n68 = case shown="True" w31 {
        tunnel: w5 -> [_ w96]
        tunnel: w25 -> [_ w102]
        tunnel: w24 -> [_ w99]
        tunnel: w5 -> [_ w97]
        frame False {
        }
        frame True {
          n69 = Unbundle By Name(w96) -> ("Loading Com Port.FFx(N)"=w106:refnum<vi>)
          n70 = Less?(x=w99, y=3.0) -> (x < y?=w98:bool)
          n71 = property class="Arr (strict)"(reference=w106) -> (reference out=w104:refnum<vi>, error out=w105:errorcluster, "Value"=w103:dbl[])  [unwired: 1 in]
          n72 = case shown="True" w98 {
            tunnel: w97 -> [_ w109]
            frame False {
            }
            frame True {
              n73 = Unbundle By Name(w109) -> ("Loading Com Port.Load Cell Temp"=w112:refnum<vi>)
              n74 = local write "Load Comflg"(FALSE ("Load Comflg")) -> ()
              n75 = property class="Bool (strict)"(reference=w112, "Value"=TRUE) -> (reference out=w110:refnum<vi>, error out=w111:errorcluster)  [unwired: 1 in]
              n76 = Close Reference(reference=w110, error in (no error)=w111) -> ()  [unwired: 1 out]
            }
          }
          n77 = Close Reference(reference=w104, error in (no error)=w105) -> ()  [unwired: 1 out]
          n78 = call-poly <vilib>:"Mean.vi"("X"=w103) -> ("mean"=w101:dbl)  [unwired: 1 out]
          n79 = case shown="True" w102 {
            tunnel: w101 -> [w113 w123]
            tunnel: w99 -> [w116 _]
            tunnel: w96 -> [_ w121]
            tunnel: w96 -> [_ w122]
            frame False {
              n80 = Less?(x=w116, y=5.0) -> (x < y?=w114:bool)
              n81 = case shown="True" w114 {
                tunnel: w113 -> [_ w118]
                frame False {
                }
                frame True {
                  n82 = Not A Number/Path/Refnum?(number/path/refnum=w118) -> (NaN/Path/Refnum?=w120:bool)
                  n83 = Select(t=1.0, s=w120, f=w118) -> (s? t:f=→"OLD VAL":dbl)
                }
              }
            }
            frame True {
              n84 = stacked-sequence {
                tunnel: w123 -> [w140 _]
                tunnel: w122 -> [w125 w213]
                tunnel: w121 -> [w124 _]
                frame #0 {
                  n85 = Unbundle By Name(w125) -> ("Loading.Warning"=w134:refnum<vi>)
                  n86 = Unbundle By Name(w124) -> ("Loading.DecaForce COM Status"=w138:refnum<vi>)
                  n87 = local read "OLD VAL"() -> (w141:dbl)
                  n88 = Unbundle By Name(w124) -> ("Loading Com Port.model"=w127:refnum<vi>)
                  n89 = Not Equal?(x=w141, y=w140) -> (x != y?=w139:bool)
                  n90 = property class="TabCtl (strict)"(reference=w134, "Visible"=TRUE) -> (reference out=w132:refnum<vi>, error out=w133:errorcluster)  [unwired: 1 in]
                  n91 = Not(x=w139) -> (.not. x?=w130:bool)
                  n92 = property class="Bool (strict)"(reference=w138, "Visible"=TRUE) -> (reference out=w136:refnum<vi>, error out=w137:errorcluster)  [unwired: 1 in]
                  n93 = property class="Str"(reference=w127) -> (reference out=w129:refnum<vi>, error out=w128:errorcluster, "Value"=w126:string)  [unwired: 1 in]
                  n94 = Close Reference(reference=w132, error in (no error)=w133) -> ()  [unwired: 1 out]
                  n95 = Close Reference(reference=w129, error in (no error)=w128) -> ()  [unwired: 1 out]
                  n96 = Close Reference(reference=w136, error in (no error)=w137) -> ()  [unwired: 1 out]
                  n97 = case shown="False" w130 {
                    tunnel: w126 -> [w146 _]
                    tunnel: w125 -> [w144 w200]
                    tunnel: w124 -> [w143 _]
                    frame False {
                      n98 = Match True/False String(2:"#####" ("true string"), 3:"HPS-FT120" ("true string"), 4:w146) -> (0:w145:bool)  [unwired: 1 out]
                      n99 = Match True/False String(2:"#####" ("true string"), 3:"HPS-FT060E" ("true string"), 4:w146) -> (0:w142:bool)  [unwired: 1 out]
                      n100 = case shown="True" w145 {
                        tunnel: w144 -> [_ w178]
                        frame False {
                        }
                        frame True {
                          w176 = T2."Disabled and Grayed Out" ("Disabled")
                          n101 = Unbundle By Name(w178) -> ("Loading.DecaForce"=w186:refnum<vi>)
                          n102 = Unbundle By Name(w178) -> ("Loading.MicroForce"=w180:refnum<vi>)
                          n103 = Unbundle By Name(w178) -> ("Loading.KiloForce"=w182:refnum<vi>)
                          n104 = Unbundle By Name(w178) -> ("Loading.SSP 0.75"=w188:refnum<vi>)
                          n105 = Unbundle By Name(w178) -> ("Loading.SSP 0.3"=w196:refnum<vi>)
                          n106 = Unbundle By Name(w178) -> ("Loading.SSP 0.5"=w193:refnum<vi>)
                          n107 = property class="Bool (strict)"(reference=w193, "Visible"=TRUE) -> (reference out=w191:refnum<vi>, error out=w192:errorcluster)  [unwired: 1 in]
                          n108 = property class="Bool (strict)"(reference=w196, "Visible"=TRUE) -> (reference out=w198:refnum<vi>, error out=w197:errorcluster)  [unwired: 1 in]
                          n109 = property class="Bool (strict)"(reference=w188, "Visible"=TRUE) -> (reference out=w190:refnum<vi>, error out=w189:errorcluster)  [unwired: 1 in]
                          n110 = property class="Bool (strict)"(reference=w186, "DisabledEnum"=w176) -> (reference out=w184:refnum<vi>, error out=w185:errorcluster)  [unwired: 1 in]
                          n111 = property class="Bool (strict)"(reference=w182, "DisabledEnum"=T2."Enabled" ("Disabled")) -> (reference out=w181:refnum<vi>, error out=w183:errorcluster)  [unwired: 1 in]
                          n112 = property class="Bool (strict)"(reference=w180, "DisabledEnum"=w176) -> (reference out=w175:refnum<vi>, error out=w179:errorcluster)  [unwired: 1 in]
                          n113 = Close Reference(reference=w191, error in (no error)=w192) -> ()  [unwired: 1 out]
                          n114 = Close Reference(reference=w198, error in (no error)=w197) -> ()  [unwired: 1 out]
                          n115 = Close Reference(reference=w190, error in (no error)=w189) -> ()  [unwired: 1 out]
                          n116 = Close Reference(reference=w184, error in (no error)=w185) -> ()  [unwired: 1 out]
                          n117 = Close Reference(reference=w181, error in (no error)=w183) -> ()  [unwired: 1 out]
                          n118 = Close Reference(reference=w175, error in (no error)=w179) -> ()  [unwired: 1 out]
                        }
                      }
                      n119 = case shown="True" w142 {
                        tunnel: w143 -> [_ w154]
                        frame False {
                        }
                        frame True {
                          w152 = T2."Disabled and Grayed Out" ("Disabled")
                          n120 = Unbundle By Name(w154) -> ("Loading.DecaForce"=w162:refnum<vi>)
                          n121 = Unbundle By Name(w154) -> ("Loading.MicroForce"=w156:refnum<vi>)
                          n122 = Unbundle By Name(w154) -> ("Loading.KiloForce"=w158:refnum<vi>)
                          n123 = Unbundle By Name(w154) -> ("Loading.SSP 0.75"=w164:refnum<vi>)
                          n124 = Unbundle By Name(w154) -> ("Loading.SSP 0.3"=w172:refnum<vi>)
                          n125 = Unbundle By Name(w154) -> ("Loading.SSP 0.5"=w169:refnum<vi>)
                          n126 = property class="Bool (strict)"(reference=w169, "Visible"=TRUE) -> (reference out=w167:refnum<vi>, error out=w168:errorcluster)  [unwired: 1 in]
                          n127 = property class="Bool (strict)"(reference=w172, "Visible"=TRUE) -> (reference out=w174:refnum<vi>, error out=w173:errorcluster)  [unwired: 1 in]
                          n128 = property class="Bool (strict)"(reference=w164, "Visible"=TRUE) -> (reference out=w166:refnum<vi>, error out=w165:errorcluster)  [unwired: 1 in]
                          n129 = property class="Bool (strict)"(reference=w162, "DisabledEnum"=T2."Enabled" ("Disabled")) -> (reference out=w160:refnum<vi>, error out=w161:errorcluster)  [unwired: 1 in]
                          n130 = property class="Bool (strict)"(reference=w158, "DisabledEnum"=w152) -> (reference out=w157:refnum<vi>, error out=w159:errorcluster)  [unwired: 1 in]
                          n131 = property class="Bool (strict)"(reference=w156, "DisabledEnum"=w152) -> (reference out=w153:refnum<vi>, error out=w155:errorcluster)  [unwired: 1 in]
                          n132 = Close Reference(reference=w167, error in (no error)=w168) -> ()  [unwired: 1 out]
                          n133 = Close Reference(reference=w174, error in (no error)=w173) -> ()  [unwired: 1 out]
                          n134 = Close Reference(reference=w166, error in (no error)=w165) -> ()  [unwired: 1 out]
                          n135 = Close Reference(reference=w160, error in (no error)=w161) -> ()  [unwired: 1 out]
                          n136 = Close Reference(reference=w157, error in (no error)=w159) -> ()  [unwired: 1 out]
                          n137 = Close Reference(reference=w153, error in (no error)=w155) -> ()  [unwired: 1 out]
                        }
                      }
                    }
                    frame True {
                      w199 = T2."Disabled and Grayed Out" ("Disabled")
                      n138 = Unbundle By Name(w200) -> ("Loading.DecaForce"=w209:refnum<vi>)
                      n139 = Unbundle By Name(w200) -> ("Loading.MicroForce"=w204:refnum<vi>)
                      n140 = Unbundle By Name(w200) -> ("Loading.KiloForce"=w206:refnum<vi>)
                      n141 = property class="Bool (strict)"(reference=w209, "DisabledEnum"=w199) -> (reference out=w201:refnum<vi>, error out=w208:errorcluster)  [unwired: 1 in]
                      n142 = property class="Bool (strict)"(reference=w206, "DisabledEnum"=w199) -> (reference out=w205:refnum<vi>, error out=w207:errorcluster)  [unwired: 1 in]
                      n143 = property class="Bool (strict)"(reference=w204, "DisabledEnum"=w199) -> (reference out=w202:refnum<vi>, error out=w203:errorcluster)  [unwired: 1 in]
                      n144 = Close Reference(reference=w201, error in (no error)=w208) -> ()  [unwired: 1 out]
                      n145 = Close Reference(reference=w205, error in (no error)=w207) -> ()  [unwired: 1 out]
                      n146 = Close Reference(reference=w202, error in (no error)=w203) -> ()  [unwired: 1 out]
                    }
                  }
                }
                frame #1 {
                  n147 = Unbundle By Name(w213) -> ("Loading.com 3"=w215:refnum<vi>)
                  n148 = property class="Bool (strict)"(reference=w215, "Value"=FALSE) -> (reference out=w212:refnum<vi>, error out=w214:errorcluster)  [unwired: 1 in]
                  n149 = Close Reference(reference=w212, error in (no error)=w214) -> ()  [unwired: 1 out]
                  "Load Comflg" <- TRUE ("Load Comflg")
                }
              }
            }
          }
        }
      }
    }
    frame Error {
    }
  }
  "error out" <- w1
